vi "Load User Apps.vi"(8 "error in (no error)":errorcluster, 11 "picoG in":refnum<class "picoG.lvclass">) -> (0 "error out":errorcluster, 3 "picoG out":refnum<class "picoG.lvclass">)   [LabVIEW 2020, in "PicoG-App.lvlib" / "picoG.lvclass"]
uses:
  picoG.lvclass
  picoG.lvclass/picoG.ctl
  App Watcher/App Watcher.lvclass
  ViaApp/ViaApp.lvclass
  AppListPanel/AppListPanel.lvclass
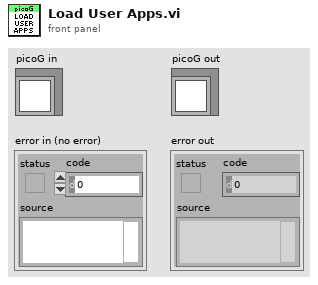
[diagram p1: front panel]
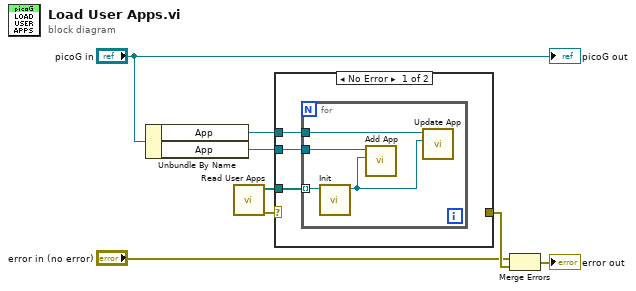
[diagram p0: block diagram]
diagram:
  n1 = Unbundle By Name("picoG in") -> ("App"=w1:refnum<class "AppListPanel.lvclass">, "App"=w6:refnum<class "App Watcher.lvclass">)
  n2 = call "Read User Apps.vi"() -> ("error out"=w8:errorcluster, "User App Paths"=w7:path[])  [unwired: 10 in]
  n3 = case shown="No Error" w8 {
    selector: w8 -> [_ w16]
    tunnel: w7 -> [w10 _]
    tunnel: w6 -> [w11 _]
    tunnel: [_ w16] -> w4
    tunnel: w1 -> [w9 _]
    frame No Error {
      n4 = for {
        tunnel: w11 -> [w15]
        tunnel: w10 -> [w14] mode=indexing
        tunnel: w9 -> [w13]
        n5 = call "Init.vi"("Path"=w14) -> ("ViaApp out"=w12:refnum<class "ViaApp.lvclass">)  [unwired: 9 in, 1 out]
        n6 = call "Add App.vi"("ViaApp"=w12, "App Watcher in"=w15) -> ()  [unwired: 8 in, 2 out]
        n7 = call "Update App.vi"("ViaApp"=w12, "AppListPanel in"=w13) -> ()  [unwired: 8 in, 2 out]
      }
    }
    frame Error {
    }
  }
  n8 = Merge Errors("error in (no error)", w4) -> (→"error out":errorcluster)
  "picoG out" <- "picoG in"
